vi "Manipulator Controller.vi"   [LabVIEW 2018]
uses:
  <vilib>/Rock Robotics/WPI/Joystick/WPI_JoystickDeviceEnum.ctl
  Manipulator Controller Global.vi
types:
  T1 = typedef "WPI_JoystickDeviceEnum.ctl" = enum16{"USB 0", "USB 1", "USB 2", "USB 3", "USB 4", "USB 5"}
  T2 = typedef "WPI_JoystickDevRef.ctl" = cluster{"Device":T1}
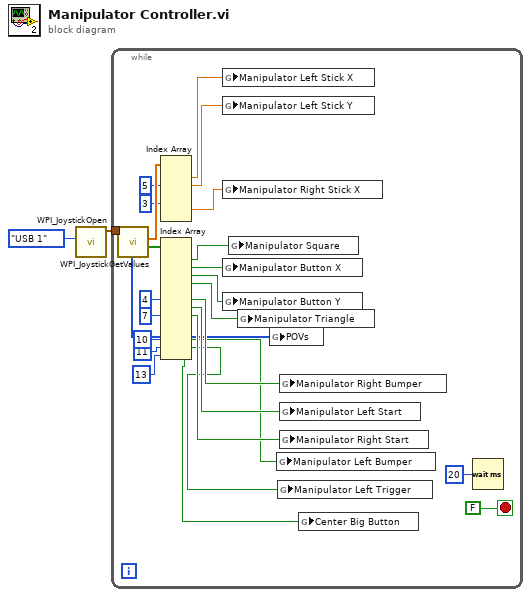
[diagram p0: block diagram]
diagram:
  n1 = call <vilib>:"WPI_JoystickOpen.vi"("JoystickDevice"=WPI_JoystickDeviceEnum."USB 1") -> ("JoystickDevRef"=w1:T2)  [unwired: 10 in]
  n2 = while {
    tunnel: w1 -> [w28]
    stop <- FALSE stop-if-true
    n3 = call <vilib>:"WPI_JoystickGetValues.vi"("JoystickDevRef"=w28) -> ("Buttons"=w26:bool[], "Axes"=w27:dbl[], "POVs"=w10:i16[])  [unwired: 6 in, 2 out]
    n4 = Index Array(array=w27, index #2=5 ("index"), index #4=3 ("index")) -> (element #1=w25:dbl, element #2=w24:dbl, element #5=w23:dbl)  [unwired: 4 in, 3 out]
    n5 = Index Array(array=w26, index #6=4 ("index"), index #8=7 ("index"), index #11=10 ("index"), index #12=11 ("index"), index #13=13 ("index")) -> (element #1=w22:bool, element #2=w21:bool, element #3=w20:bool, element #4=w9:bool, element #6=w19:bool, element #7=w18:bool, element #8=w17:bool, element #11=w7:bool, element #12=w5:bool, element #13=w3:bool)  [unwired: 8 in, 3 out]
    n6 = global write "Manipulator Controller Global.vi" "Manipulator Left Stick X"(w25) -> ()
    n7 = global write "Manipulator Controller Global.vi" "Manipulator Left Stick Y"(w24) -> ()
    n8 = global write "Manipulator Controller Global.vi" "Manipulator Right Stick X"(w23) -> ()
    n9 = global write "Manipulator Controller Global.vi" "Manipulator Button X"(w21) -> ()
    n10 = global write "Manipulator Controller Global.vi" "Manipulator Button Y"(w20) -> ()
    n11 = global write "Manipulator Controller Global.vi" "Manipulator Square"(w22) -> ()
    n12 = global write "Manipulator Controller Global.vi" "Manipulator Triangle"(w9) -> ()
    n13 = global write "Manipulator Controller Global.vi" "POVs"(w10) -> ()
    n14 = global write "Manipulator Controller Global.vi" "Manipulator Left Bumper"(w7) -> ()
    n15 = global write "Manipulator Controller Global.vi" "Manipulator Left Trigger"(w5) -> ()
    n16 = global write "Manipulator Controller Global.vi" "Manipulator Right Bumper"(w19) -> ()
    n17 = global write "Manipulator Controller Global.vi" "Manipulator Left Start"(w18) -> ()
    n18 = global write "Manipulator Controller Global.vi" "Manipulator Right Start"(w17) -> ()
    n19 = global write "Manipulator Controller Global.vi" "Center Big Button"(w3) -> ()
    n20 = Wait (ms)(milliseconds to wait=u32 20) -> ()  [unwired: 1 out]
  }
